vi "Stop Target.vi"(7 "Target Ident":string, 8 "Error In":errorcluster, 11 "reference in":refnum<class "Measure and Stimulus Subsystems.lvclass">) -> (0 "Error Out":errorcluster, 3 "reference out":refnum<class "Measure and Stimulus Subsystems.lvclass">)   [LabVIEW 2023, in "HAL GOOP4.lvlib" / "Measure and Stimulus Subsystems.lvclass"]
uses:
  Measure and Stimulus Subsystems.lvclass
  Measure and Stimulus Subsystems.lvclass/Measure and Stimulus Subsystems.ctl
  Virt Instrument Base/Virt Instr Base.lvclass
  <vilib>/Utility/error.llb/Error Cluster From Error Code.vi
  <vilib>/ErrorRing/Error Ring.xnode
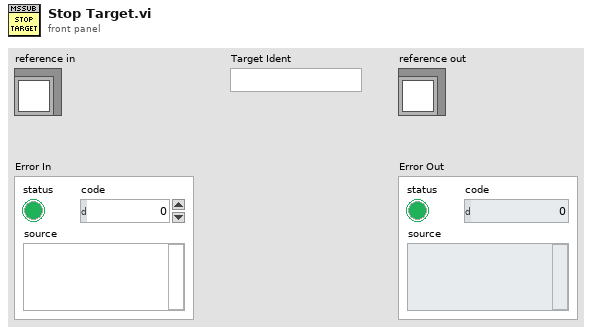
[diagram p1: front panel]
types:
  T1 = typedef "HAL GOOP4.lvlib/Measure and Stimulus Subsystems.lvclass/ObjectAttributes.ctl" = cluster{"Virt Instr":map{string, refnum<class "Virt Instr Base.lvclass">}, "Phys Instr":map{string, cluster{"Instrument Base":refnum<class "Instr Base.lvclass">, "Ref Count":u8}}}
  T2 = map{string, refnum<class "Virt Instr Base.lvclass">}
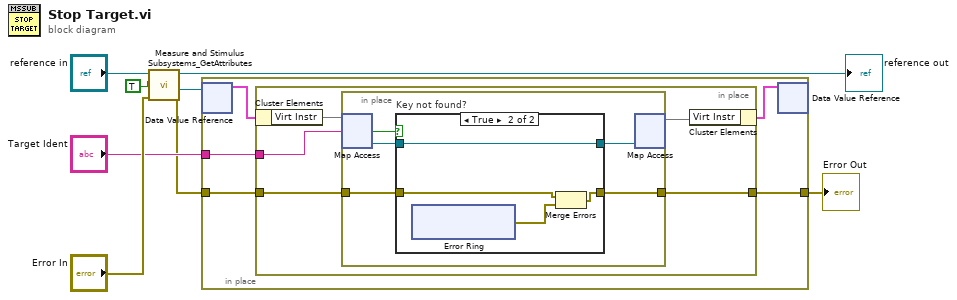
[diagram p0: block diagram]
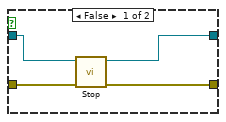
[diagram p2: hidden frame]
diagram:
  n1 = call "Measure and Stimulus Subsystems_GetAttributes.vi"("Error In"="Error In", "OnlyGetDvrReference(False)"=TRUE, "reference in"="reference in") -> ("Error Out"=w3:errorcluster, "DataRef"=w1:refnum<data-value>, "reference out"=→"reference out":refnum<class "Measure and Stimulus Subsystems.lvclass">)  [unwired: 5 in, 1 out]
  n2 = in-place {
    in-place-border: [w13] -> w5
    in-place-border: "Target Ident" -> [w12]
    in-place-border: w3 -> [w11]
    n3 = in-place-dvr #1(w1) -> (w10:T1)  [unwired: 1 out]
    n4 = in-place {
      in-place-border: [w18] -> w13
      in-place-border: w12 -> [w17]
      in-place-border: w11 -> [w16]
      n5 = in-place-cluster #2(w10) -> ("Virt Instr"=w15:T2)
      n6 = in-place {
        in-place-border: w16 -> [w21]
        in-place-border: [w19] -> w18
        n7 = in-place-map #3(w15, w17) -> (w22:refnum<class "Virt Instr Base.lvclass">, w23:bool)  [unwired: 1 in]
        n8 = case "Key not found?" shown="True" w23 {
          tunnel: w22 -> [w24 w28]
          tunnel: w21 -> [w27 w29]
          tunnel: [w25 w28] -> w20
          tunnel: [w26 w31] -> w19
          frame False {
            n9 = call "Stop.vi"("error in (no error)"=w27, "Virt Instr Base in"=w24) -> ("error out"=w26:errorcluster, "Virt Instr Base out"=w25:refnum<class "Virt Instr Base.lvclass">)  [unwired: 8 in]
          }
          frame True {
            n10 = xnode "Error Ring"() -> ("error out"=w30:errorcluster)
            n11 = Merge Errors(w29, w30) -> (w31:errorcluster)
          }
        }
        n12 = in-place-map #3(w20) -> (w14:T2)  [unwired: 1 in, 2 out]
      }
      n13 = in-place-cluster #2("Virt Instr"=w14) -> (w9:T1)
    }
    n14 = in-place-dvr #1(w9) -> ()  [unwired: 2 out]
  }
  "Error Out" <- w5
